vi "syslog_PublishArray.vi"(9 "Time Target (s)":dbl=1.0, 10 "Input Array In":dbl[](array[numeric]), 11 "Output Array In":dbl[](array[numeric])) -> (2 "Input Array Out":dbl[](array[numeric]), 3 "Output Array Out":dbl[](array[numeric]))   [LabVIEW 2016, in "Scan Engine Custom Device.lvlib"]
uses:
  Scan Engine Custom Device.lvlib
  <vilib>/NI/syslog/_subVIs/TypeDefs/syslog_severity_codes.ctl
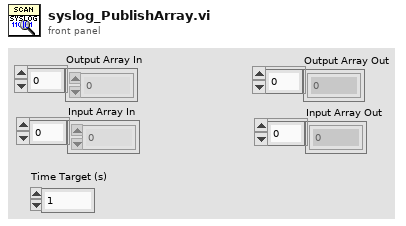
[diagram p1: front panel]
types:
  T1 = typedef "syslog_severity_codes.ctl" = enum16{"emergency", "alert", "critical", "error", "warning", "notice", "info", "debug"}
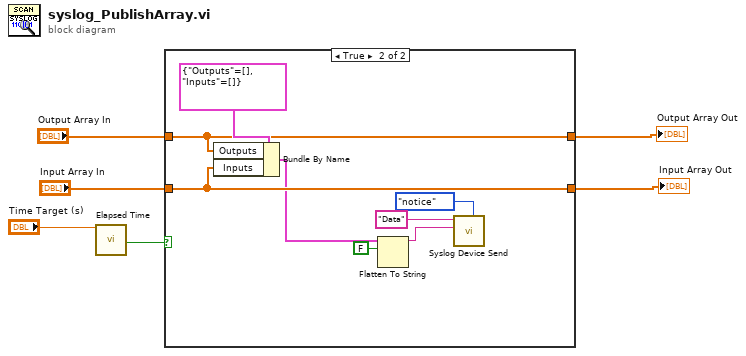
[diagram p0: block diagram]
diagram:
  n1 = call "Elapsed Time"("Time Target (s)"="Time Target (s)") -> ("Time has Elapsed"=w4:bool)  [unwired: 11 in, 7 out]
  n2 = case shown="True" w4 {
    tunnel: "Output Array In" -> [w8 w15]
    tunnel: "Input Array In" -> [w7 w14]
    tunnel: [w8 w15] -> w2
    tunnel: [w7 w14] -> w1
    frame False {
    }
    frame True {
      n3 = Bundle By Name(cluster=cluster{"Outputs":dbl[], "Inputs":dbl[]} {"Outputs"=[], "Inputs"=[]} ("Cluster"), "Outputs"=w15, "Inputs"=w14) -> (w11:cluster{"Outputs":dbl[], "Inputs":dbl[]})
      n4 = Flatten To String(anything=w11, prepend array or string size? (T)=FALSE) -> (data string=w10:string)  [unwired: 2 in, 2 out]
      n5 = call <vilib>:"Syslog Device Send.vi"("Severity Code (error)"=syslog_severity_codes."notice", "Message Content"=w10, "Message Tag"="Data") -> ()  [unwired: 7 in, 2 out]
    }
  }
  "Output Array Out" <- w2
  "Input Array Out" <- w1
